vi "Mass_2_2.vi"() -> ()   [LabVIEW 2020]
uses:
  Support/Controls/Cmd_Mouse Popup.ctl
  Support/Controls/Clst_Initialize Input.ctl
  Support/Controls/Clst_Result inspec.ctl
  Support/Controls/Cmd_Var Data IO.ctl
  Variables/Global_Cal Info.vi
  <vilib>/express/express arith-compare/Formula/XNode/ExpressFormulaBlockNode.xnode
panel:
  in  "일괄\n변경":bool=TRUE
  in  "추가문자열":string
  in  "추가단위":string(combo)="mg" caption="단위"
  in  "호칭":string
  out "환산값":string caption="환산값 (g)"
  in  "분동등급":string(combo)
  out "적용?":bool
  in  "다음 버튼":bool
  in  "이전 버튼":bool
  in  "제거":bool
  in  "적용":bool
  in  "추가명목값":string caption="명목값"
  in  "추가":bool
  out "분해능":string caption="저울분해능 (g)"
  out "Data Out":string[][](table)
  out "단위":string
  out "명목질량":string
  in  "기기번호":string
  out "명목값":string
  in  "편심오차":string[][](table) caption="4. 저울 편심오차 시험"
  in  "시험분동밀도":string="8000" caption="분동밀도 (kg/㎤)"
  out "감도분동":string
  out "X=S-T":string[][](table)
  out "공기밀도":string
  out "Header2":string[][](table)
  in  "Measured":string[][](table) caption="3. 저울 지시값"
  out "Weight info":string[][](table) caption="2. 분동식별표기"
  out "Spec":string[][](table)
  in  "시험분동":i32(listbox)=-1
  in  "Spec 변경":bool
  out "제목":string
  out "에러 출력":errorcluster
  out "Condition":string[][](table)
  out "Atm Env":string[][](table) caption="1. 측정환경"
  out "Load?":bool
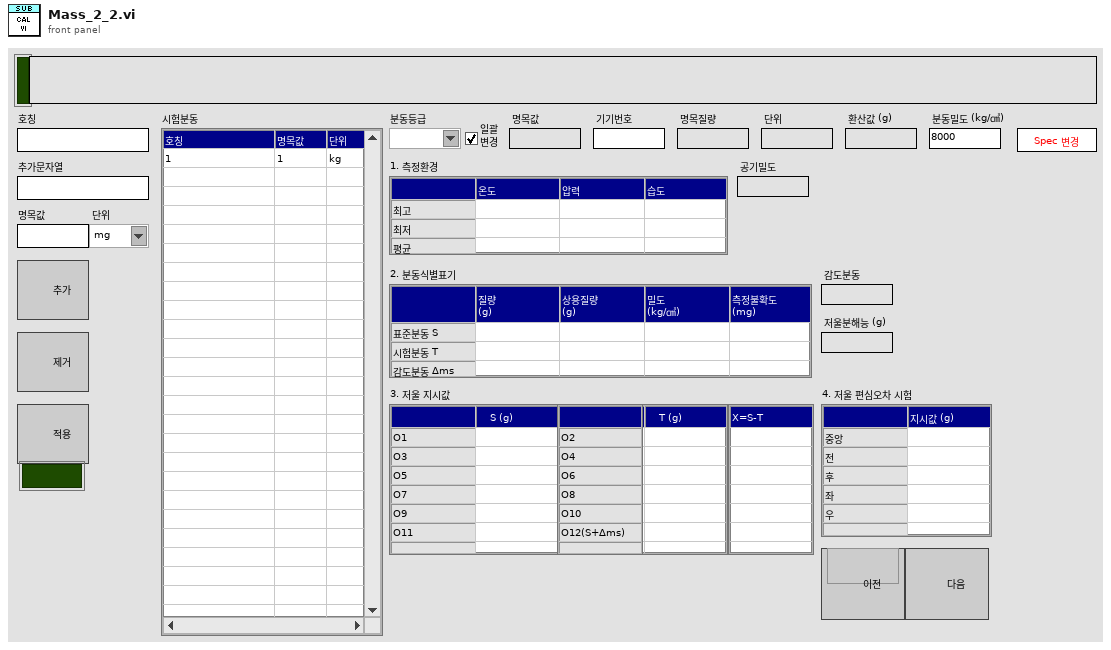
[diagram p1: front panel]
types:
  T1 = typedef "Cmd_Mouse Popup.ctl" = enum16{"활성화", "메뉴선택"}
  T2 = cluster{"Shift":bool, "Ctrl":bool, "Alt":bool, "Cmd":bool, "Opt":bool}
  T3 = typedef "Clst_Initialize Input.ctl" = cluster{"Initialize 1":cluster{"Condition":refnum<vi>[], "Spec":refnum<vi>[], "Measured":refnum<vi>[], "Resolution":refnum<vi>[], "Func_ext":string, "제목":refnum<vi>, "Measured_ADJ":refnum<vi>[]}, "Initialize 2":cluster{"문자열":refnum<vi>[], "콤보박스":refnum<vi>[], "링":refnum<vi>[], "열거형":refnum<vi>[], "테이블":refnum<vi>[], "여러열":refnum<vi>[], "디지털(DBL)":refnum<vi>[], "3D string":refnum<vi>[], "ctrl":refnum<vi>[], "boolean":refnum<vi>[]}}
  T4 = typedef "Cmd_Var Data IO.ctl" = enum16{"Condition", "Condition Default", "Condition_Temp", "Resolution", "Resolution Default", "Resolution Old", "Spec", "Spec Default", "Spec Old", "Spec Temp", "Result", "Result2", "Result3", "Result_Temp", "Result_ADJ", "Result_ADJ2", "STD1", "STD2", "STD3", "STD4", "STD5", "STD Temp", "CMC", "CMC Default"}
  T5 = typedef "Clst_Result inspec.ctl" = cluster{"분해능":string, "문자열 1":string, "문자열 2":string, "숫자형 1":i32, "숫자형 2":i32, "숫자형 3":dbl, "문자배열 1D":string[], "문자배열 2D":string[][], "문자배열 3D":string[][][], "문자배열 4D":string[][][][], "불리언 1D":bool[]}
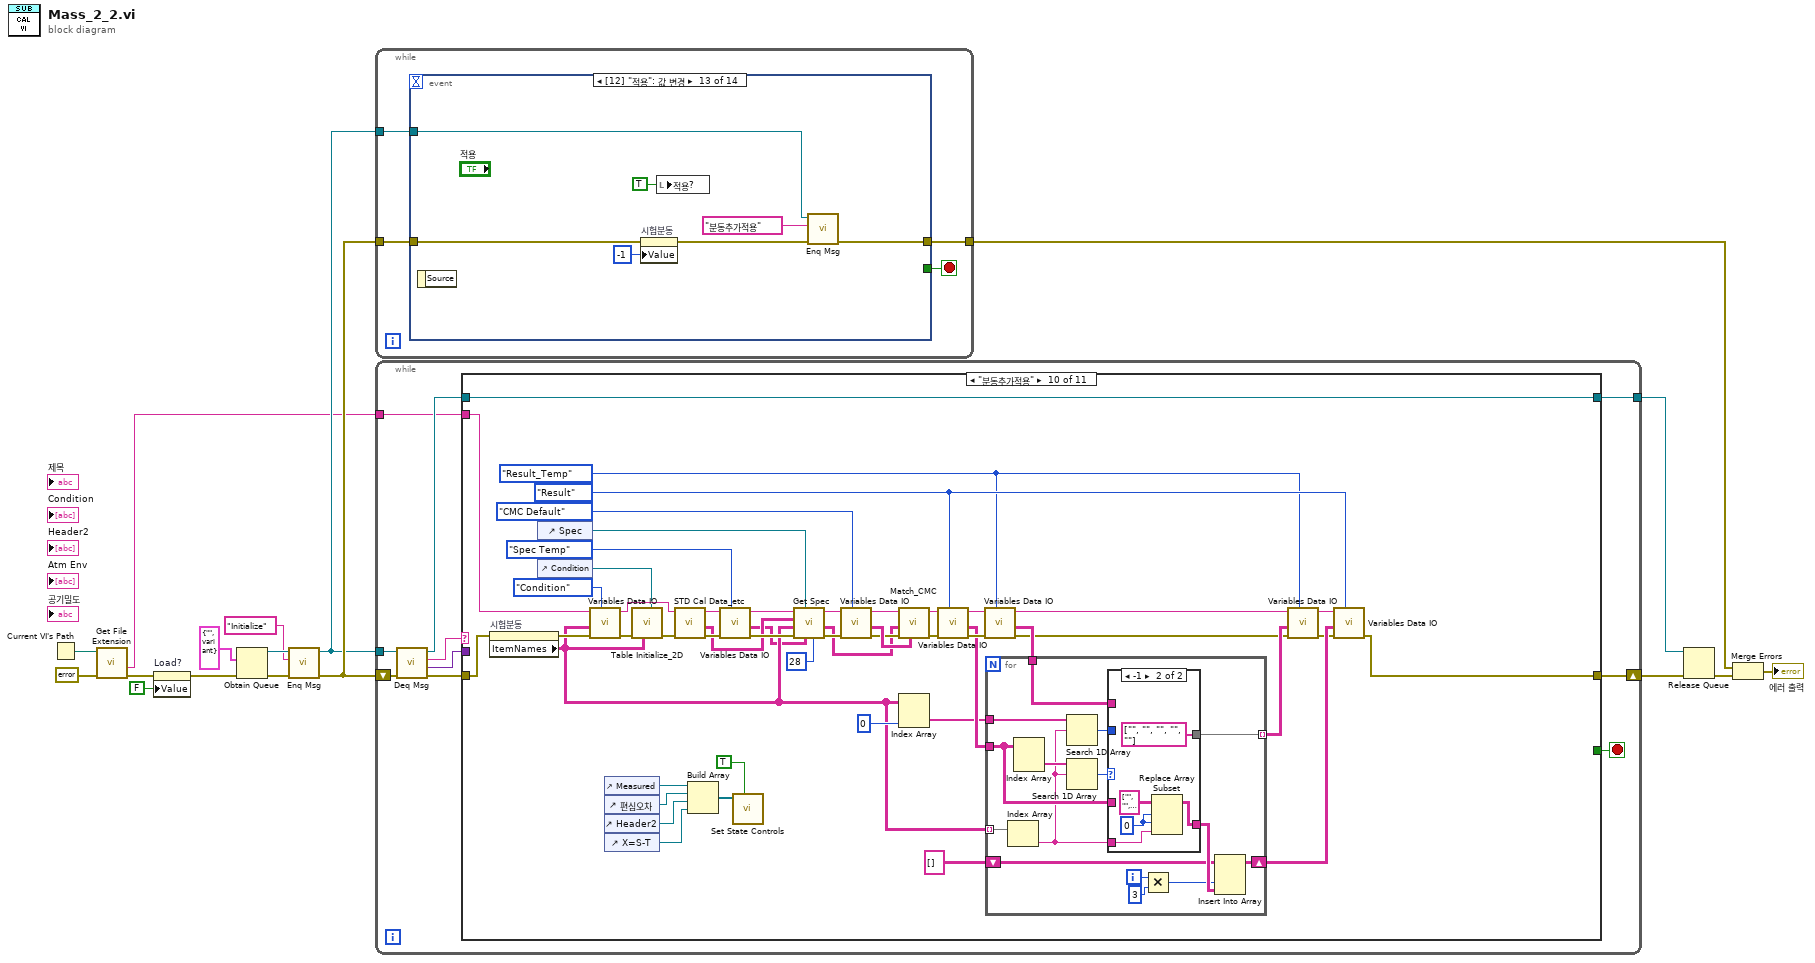
[diagram p0: block diagram]
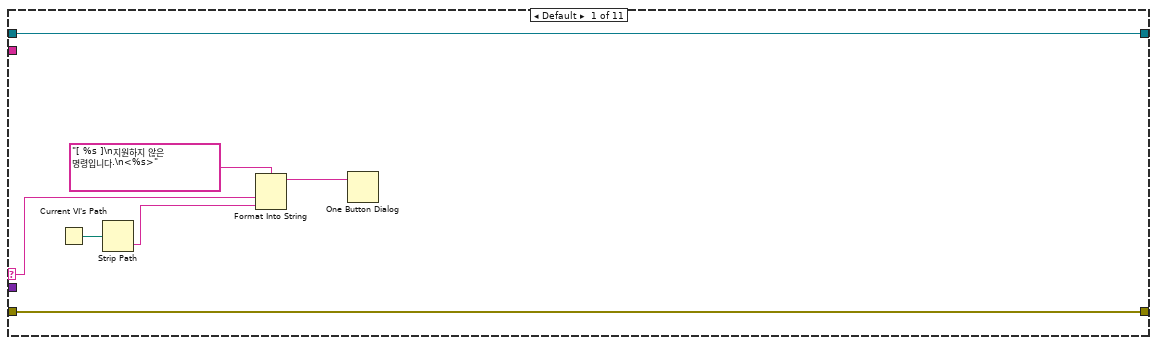
[diagram p2: hidden frame]
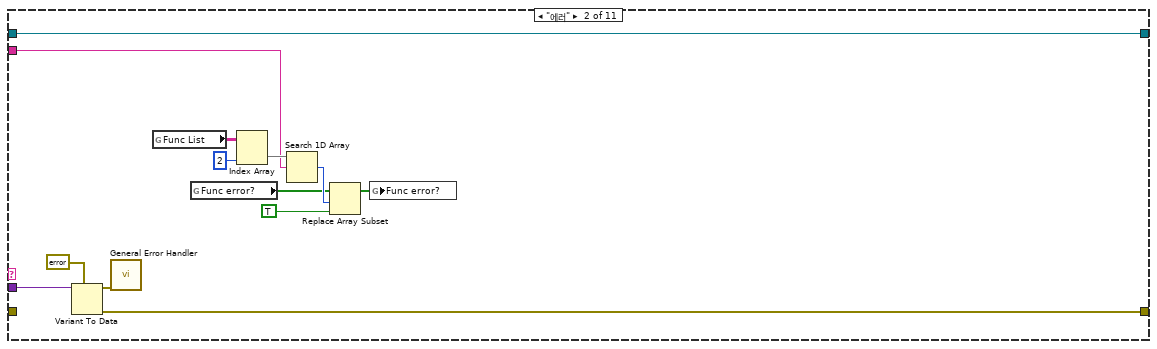
[diagram p3: hidden frame]
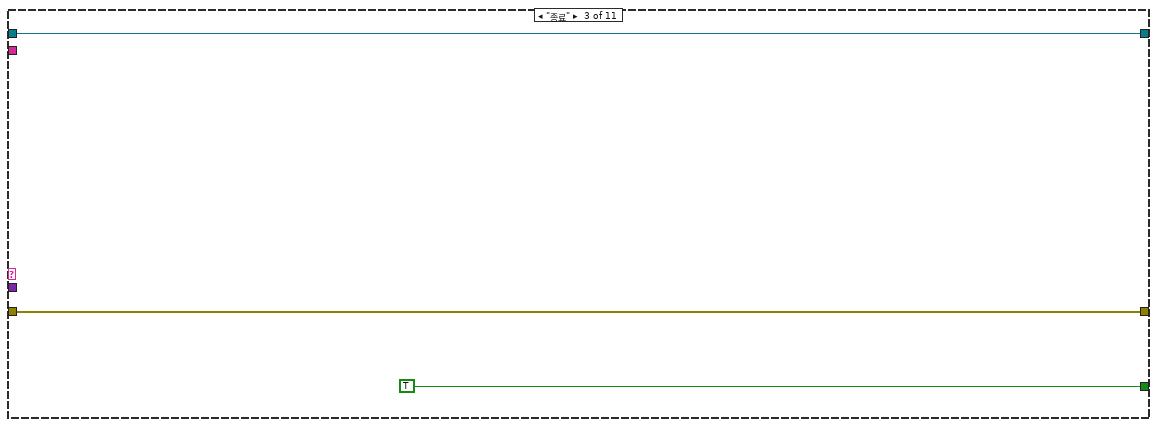
[diagram p4: hidden frame]
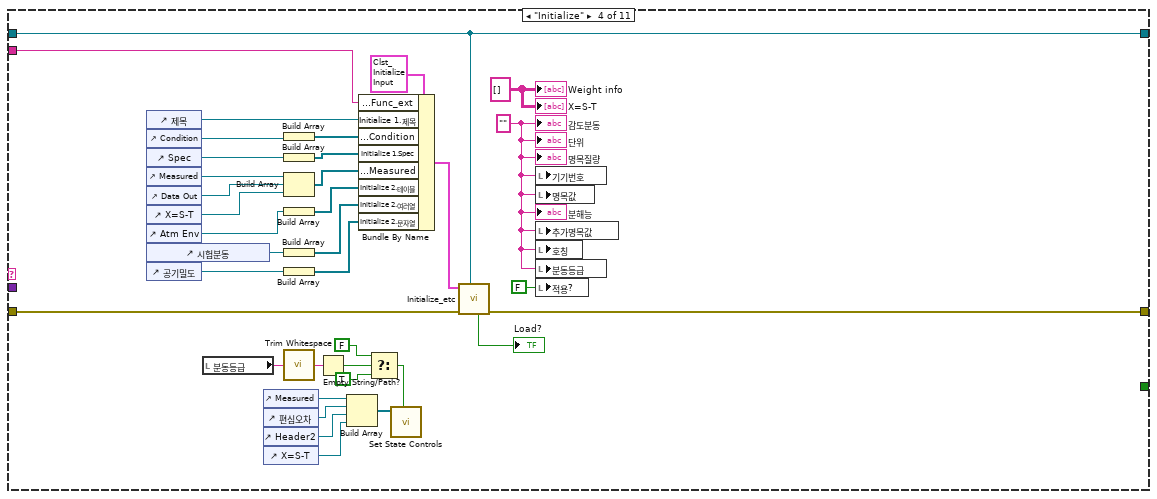
[diagram p5: hidden frame]
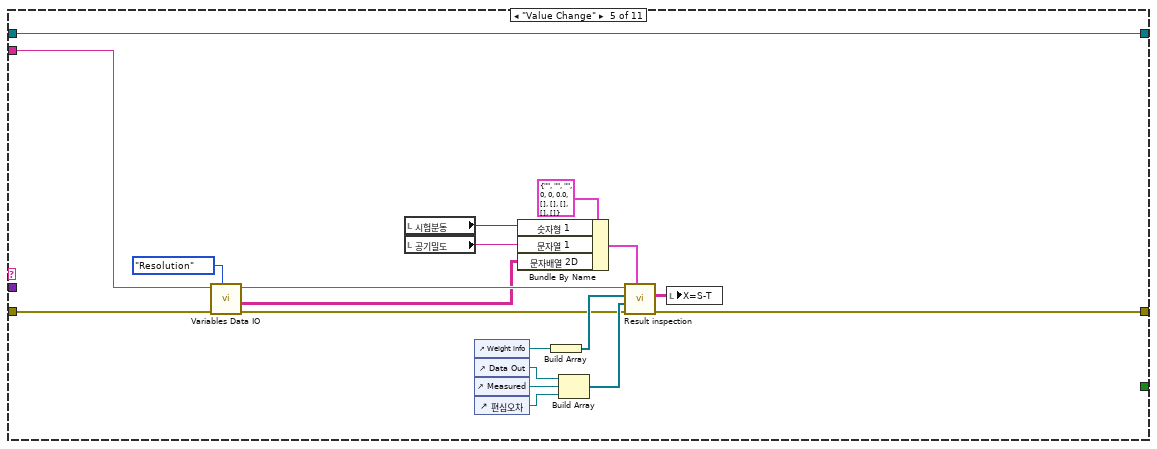
[diagram p6: hidden frame]
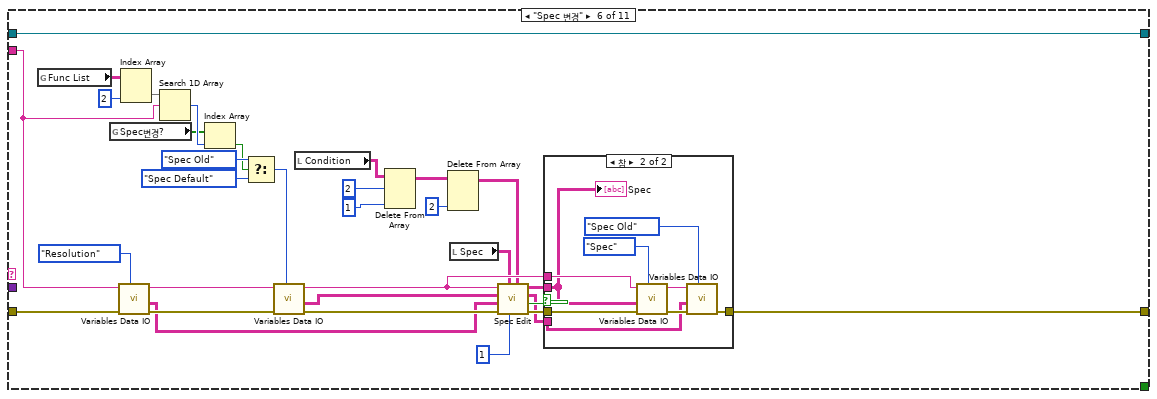
[diagram p7: hidden frame]
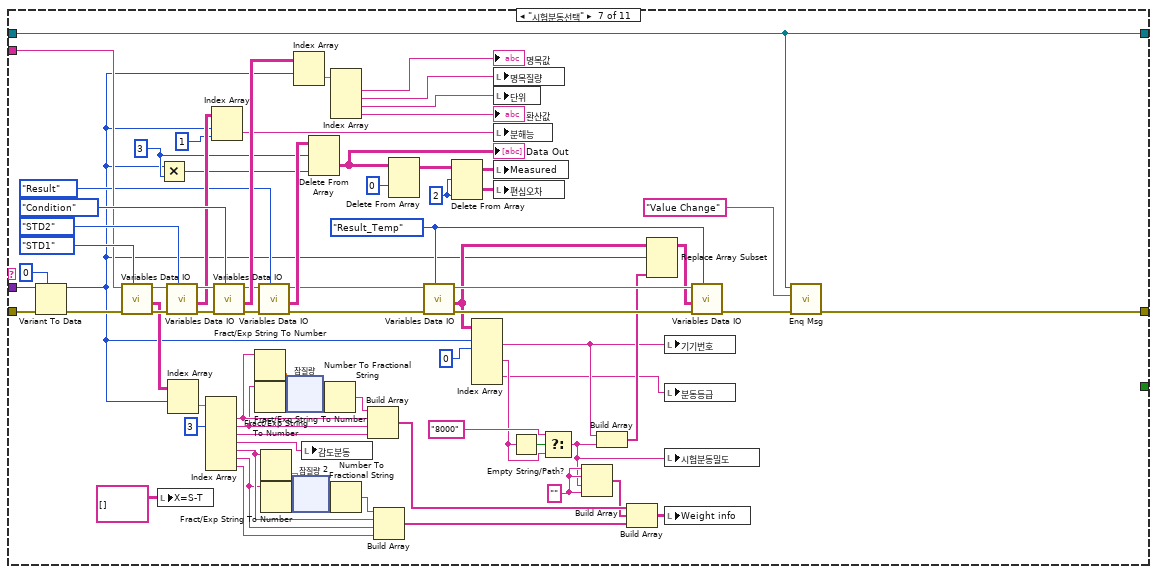
[diagram p9: hidden frame]
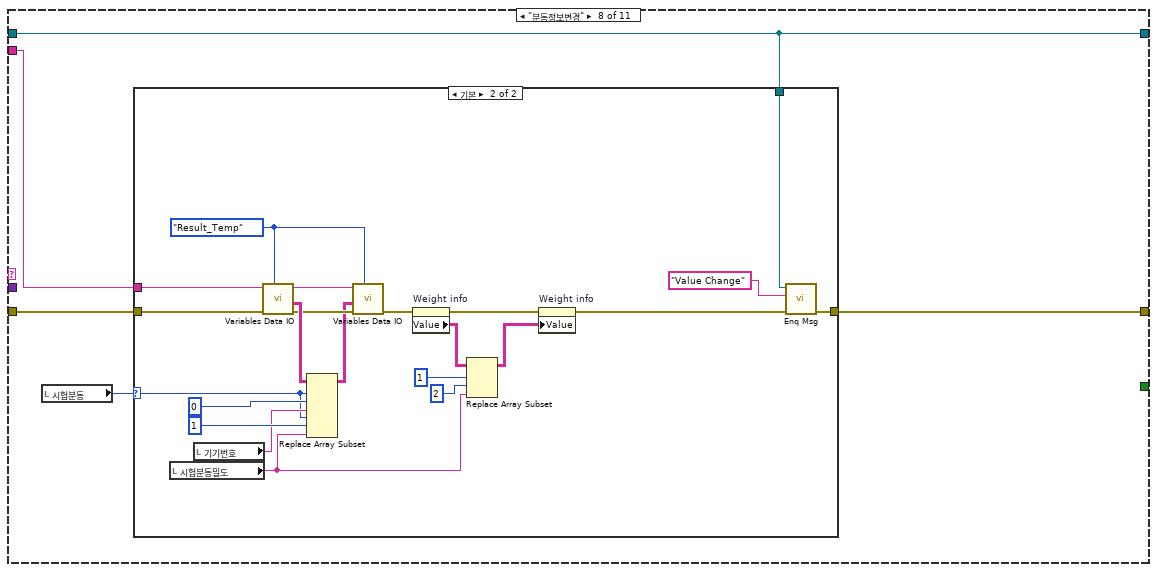
[diagram p10: hidden frame]
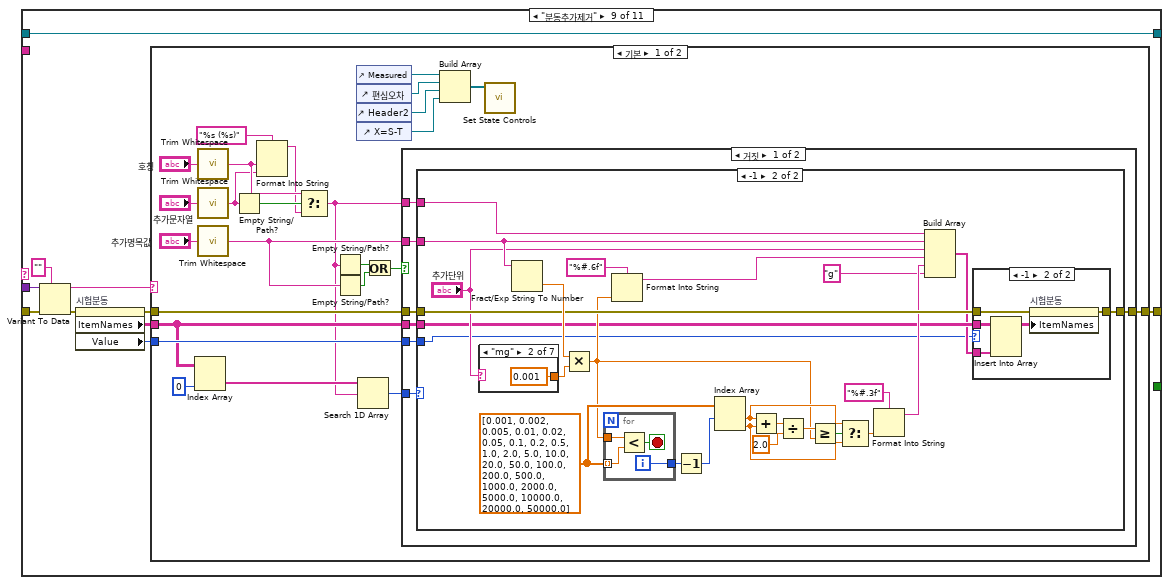
[diagram p12: hidden frame]
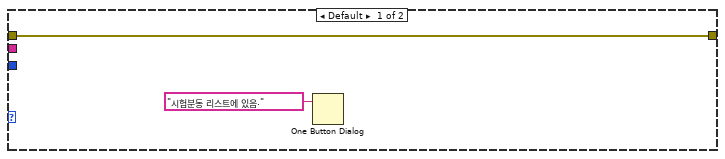
[diagram p13: hidden frame]
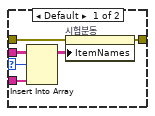
[diagram p14: hidden frame]
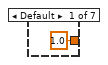
[diagram p15: hidden frame]
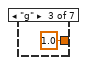
[diagram p16: hidden frame]
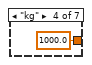
[diagram p17: hidden frame]
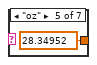
[diagram p18: hidden frame]
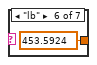
[diagram p19: hidden frame]
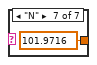
[diagram p20: hidden frame]
diagram:
  n1 = Current VI's Path() -> (path=w5:path)
  n2 = call <vilib>:"Get File Extension.vi"("error in (no error)"=errorcluster {"status"=FALSE, "code"=0, "source"=""} ("에러 상수"), "file"=w5) -> ("error out"=w3:errorcluster, "filename without extension"=w4:string)  [unwired: 5 in, 3 out]
  n3 = property on="Load?" class="Bool (엄격한)"(error in=w3, "Value"=FALSE ("Load?")) -> (error out=w2:errorcluster)  [unwired: 1 in, 1 out]
  n4 = Obtain Queue(element data type=cluster{"메세지":string, "값":variant} {"메세지"="", "값"=variant} ("Message Cluster"), error in (no error)=w2) -> (queue out=w14:refnum<queue>, error out=w16:errorcluster)  [unwired: 3 in, 1 out]
  n5 = call "Enq Msg.vi"("에러 입력(에러 없음)"=w16, "메세지"="Initialize", "큐 입력"=w14) -> ("에러 출력"=w15:errorcluster, "큐 출력"=w12:refnum<queue>)  [unwired: 7 in]
  n6 = while {
    tunnel: w15 -> [w19]
    tunnel: w12 -> [w20]
    tunnel: [w18] -> w9
    stop <- w21 stop-if-true
    n7 = event shown="[12] \"적용\": 값 변경" {
      selector: _ -> [_ _ _ _ _ _ _ _ _ _ _ _ _ _]
      dyn-events: _ -> [_ _ _ _ _ _ _ _ _ _ _ _ _ _]
      timeout: _ -> [_ _ _ _ _ _ _ _ _ _ _ _ _ _]
      tunnel: [w26 _ _ _ _ _ _ _ _ _ _ _ _ _] -> w21
      tunnel: w20 -> [w24 w29 _ w36 _ w49 w58 _ w79 w102 w117 w122 w136 w137]
      tunnel: w19 -> [w25 w30 w33 w41 w48 w51 w60 w72 w81 w96 w119 w129 w134 w139]
      tunnel: [w22 w28 w32 w35 w47 w50 w54 w72 w80 w104 w118 w121 w135 w138] -> w18
      event Panel Close? {
        w26 = TRUE ("버림?")
        n8 = event-data() -> ()  [unwired: 1 in, 1 out]
        n9 = call "Enq Msg.vi"("에러 입력(에러 없음)"=w25, "메세지"="종료", "큐 입력"=w24) -> ("에러 출력"=w22:errorcluster)  [unwired: 7 in, 1 out]
        n10 = event-data("Discard?"=w26) -> ()  [unwired: 1 in, 1 out]
      }
      event "Measured", "편심오차": Value Change {
        n11 = event-data() -> ()  [unwired: 1 in, 3 out]
        n12 = call "Enq Msg.vi"("에러 입력(에러 없음)"=w30, "메세지"="Value Change", "큐 입력"=w29) -> ("에러 출력"=w28:errorcluster)  [unwired: 7 in, 1 out]
      }
      event "Measured", "편심오차": Shortcut Menu Activation? {
        n13 = event-data() -> ("MenuRef"=w31:refnum<k9>)  [unwired: 1 in]
        n14 = call "Mouse PopUp Control.vi"("type"=Cmd_Mouse_Popup."활성화", "error in"=w33, "메뉴 참조"=w31) -> ("error out"=w32:errorcluster)  [unwired: 8 in]
        n15 = event-data() -> ()  [unwired: 2 in, 1 out]
      }
      event "Measured", "편심오차": Shortcut Menu Selection (User) {
        n16 = event-data() -> ("CtlRef"=w39:refnum<vi>, "ItemTag"=w40:string)  [unwired: 1 in]
        n17 = call "Mouse PopUp Control.vi"("type"=Cmd_Mouse_Popup."메뉴선택", "error in"=w41, "아이템 태그"=w40, "Tbl 참조 번호"=w39) -> ("error out"=w37:errorcluster)  [unwired: 7 in]
        n18 = call "Enq Msg.vi"("에러 입력(에러 없음)"=w37, "메세지"="Value Change", "큐 입력"=w36) -> ("에러 출력"=w35:errorcluster)  [unwired: 7 in, 1 out]
      }
      event "Measured", "편심오차", "Condition": Key Down; "Measured", "편심오차", "Condition": Key Repeat {
        n19 = event-data() -> ("PlatMods"=w43:T2, "ScanCode"=w46:i16, "Mods.Num Pad"=w45:bool, "CtlRef"=w44:refnum<vi>)  [unwired: 1 in]
        n20 = call "Cursor Control.vi"("플랫폼 조합키"=w43, "참조"=w44, "Num Pad"=w45, "ScanCode"=w46, "error in"=w48) -> ("error out"=w47:errorcluster)  [unwired: 5 in, 1 out]
      }
      event "Spec 변경": Value Change {
        n21 = event-data() -> ()  [unwired: 1 in, 1 out]
        n22 = call "Enq Msg.vi"("에러 입력(에러 없음)"=w51, "메세지"="Spec 변경", "큐 입력"=w49) -> ("에러 출력"=w50:errorcluster)  [unwired: 7 in, 1 out]
      }
      event "시험분동": Value Change {
        n23 = event-data() -> ()  [unwired: 1 in, 1 out]
        n24 = local read "적용?"() -> (w57:bool)
        n25 = To Variant(anything="시험분동") -> (Variant=w59:variant)
        n26 = Less Than 0?(x="시험분동") -> (x < 0?=w53:bool)
        n27 = case shown="거짓" w57 {
          tunnel: w60 -> [w66 w70]
          tunnel: [w66 w69] -> w55
          tunnel: w59 -> [_ w68]
          tunnel: w58 -> [_ w67]
          frame False {
            n28 = control-ref of="Measured"() -> (w62:refnum<vi>)
            n29 = control-ref of="편심오차"() -> (w61:refnum<vi>)
            n30 = control-ref of="Header2"() -> (w64:refnum<vi>)
            n31 = control-ref of="X=S-T"() -> (w65:refnum<vi>)
            n32 = Build Array(w62, w61, w64, w65) -> (w63:refnum<vi>[])
            n33 = call "Set State Controls.vi"("컨트롤 참조 배열 in"=w63) -> ()  [unwired: 9 in, 2 out]
          }
          frame True {
            n34 = call "Enq Msg.vi"("에러 입력(에러 없음)"=w70, "값"=w68, "메세지"="시험분동선택", "큐 입력"=w67) -> ("에러 출력"=w69:errorcluster)  [unwired: 6 in, 1 out]
          }
        }
        n35 = property on="일괄\n변경" class="Bool (엄격한)"(error in=w55, "Value"=w53) -> (error out=w54:errorcluster)  [unwired: 1 in, 1 out]
      }
      event "시험분동": Drag Ended {
        n36 = event-data() -> ()  [unwired: 1 in, 4 out]
        n37 = control-ref of="Measured"() -> (w74:refnum<vi>)
        n38 = control-ref of="편심오차"() -> (w73:refnum<vi>)
        n39 = control-ref of="Header2"() -> (w76:refnum<vi>)
        n40 = control-ref of="X=S-T"() -> (w77:refnum<vi>)
        n41 = local write "적용?"(FALSE ("적용?")) -> ()
        n42 = Build Array(w74, w73, w76, w77) -> (w75:refnum<vi>[])
        n43 = call "Set State Controls.vi"("컨트롤 참조 배열 in"=w75) -> ()  [unwired: 9 in, 2 out]
      }
      event "시험분동": Double Click {
        n44 = event-data() -> ()  [unwired: 1 in, 1 out]
        n45 = local read "적용?"() -> (w82:bool)
        n46 = case shown="거짓" w82 {
          tunnel: w81 -> [w84 w89]
          tunnel: [w86 w89] -> w80
          tunnel: w79 -> [w85 _]
          frame False {
            n47 = To Variant(anything="제거") -> (Variant=w87:variant)
            n48 = call "Enq Msg.vi"("에러 입력(에러 없음)"=w84, "값"=w87, "메세지"="분동추가제거", "큐 입력"=w85) -> ("에러 출력"=w86:errorcluster)  [unwired: 6 in, 1 out]
          }
          frame True {
          }
        }
      }
      event "이전 버튼", "다음 버튼": Value Change {
        n49 = event-data() -> ()  [unwired: 1 in, 1 out]
        n50 = property on="시험분동" class="MCListbox (엄격한)"(error in=w96) -> (error out=w95:errorcluster, "Value"=w94:i32, "ItemNames"=w93:string[][])  [unwired: 1 in, 1 out]
        n51 = Build Array("이전 버튼", "다음 버튼") -> (w99:bool[])
        n52 = Array Size(array=w93) -> (size(s)=w92:i32[])
        n53 = Boolean Array To Number(Boolean array=w99) -> (number=w98:u32)
        n54 = Index Array(array=w92) -> (element=w91:i32)  [unwired: 1 in]
        n55 = Decrement(x=w91) -> (x-1=w90:i32)
        n56 = case shown="2" w98 {
          tunnel: w94 -> [w106 w110 w116]
          tunnel: [w106 w107 w115] -> w97
          tunnel: w90 -> [_ _ w113]
          frame Default {
          }
          frame 1 {
            n57 = Less Or Equal To 0?(x=w110) -> (x <= 0?=w111:bool)
            n58 = Decrement(x=w110) -> (x-1=w109:i32)
            n59 = Select(t=0, s=w111, f=w109) -> (s? t:f=w107:i32)
          }
          frame 2 {
            n60 = Increment(x=w116) -> (x+1=w114:i32)
            n61 = Less Or Equal?(x=w114, y=w113) -> (x <= y?=w112:bool)
            n62 = Select(t=w114, s=w112, f=w116) -> (s? t:f=w115:i32)
          }
        }
        n63 = local write "시험분동"(w97) -> ()
        n64 = To Variant(anything=w97) -> (Variant=w103:variant)
        n65 = call "Enq Msg.vi"("에러 입력(에러 없음)"=w95, "값"=w103, "메세지"="시험분동선택", "큐 입력"=w102) -> ("에러 출력"=w104:errorcluster)  [unwired: 6 in, 1 out]
      }
      event "기기번호", "시험분동밀도": Value Change {
        n66 = event-data() -> ()  [unwired: 1 in, 3 out]
        n67 = call "Enq Msg.vi"("에러 입력(에러 없음)"=w119, "메세지"="분동정보변경", "큐 입력"=w117) -> ("에러 출력"=w118:errorcluster)  [unwired: 7 in, 1 out]
      }
      event "추가", "제거": Value Change {
        n68 = event-data() -> ("CtlRef"=w128:refnum<vi>)  [unwired: 1 in]
        n69 = property class="Bool"(reference=w128, error in=w129) -> (error out=w124:errorcluster, "Label.Text"=w123:string)  [unwired: 1 out]
        n70 = To Variant(anything=w123) -> (Variant=w125:variant)
        n71 = call "Enq Msg.vi"("에러 입력(에러 없음)"=w124, "값"=w125, "메세지"="분동추가제거", "큐 입력"=w122) -> ("에러 출력"=w121:errorcluster)  [unwired: 6 in, 1 out]
        "적용?" <- FALSE ("적용?")
      }
      event "적용": Value Change {
        n72 = event-data() -> ()  [unwired: 1 in, 1 out]
        n73 = property on="시험분동" class="MCListbox (엄격한)"(error in=w134, "Value"=-1 ("시험분동")) -> (error out=w132:errorcluster)  [unwired: 1 in, 1 out]
        n74 = local write "적용?"(TRUE ("적용?")) -> ()
        n75 = call "Enq Msg.vi"("에러 입력(에러 없음)"=w132, "메세지"="분동추가적용", "큐 입력"=w136) -> ("에러 출력"=w135:errorcluster)  [unwired: 7 in, 1 out]
      }
      event "분동등급": Value Change {
        n76 = event-data() -> ()  [unwired: 1 in, 3 out]
        n77 = call "Enq Msg.vi"("에러 입력(에러 없음)"=w139, "메세지"="분동등급변경", "큐 입력"=w137) -> ("에러 출력"=w138:errorcluster)  [unwired: 7 in, 1 out]
      }
    }
  }
  n78 = while {
    shift-right: [w150] -> w11
    shift-left: w15 -> [w149]
    tunnel: w12 -> [w147]
    tunnel: [w142] -> w10
    tunnel: w4 -> [w141]
    stop <- w143 stop-if-true
    n79 = call "Deq Msg.vi"("에러 입력(에러 없음)"=w149, "큐 입력"=w147) -> ("에러 출력"=w148:errorcluster, "값"=w144:variant, "메세지"=w146:string, "큐 출력"=w145:refnum<queue>)  [unwired: 6 in]
    n80 = case shown="\"분동추가적용\"" w146 {
      selector: w146 -> [w153 _ _ _ _ _ _ _ _ _ _]
      tunnel: w148 -> [w157 _ w173 w178 w214 w254 w347 w372 w403 w525 w582]
      tunnel: [w157 w167 w173 w196 w224 w258 w274 w371 w397 w514 w577] -> w150
      tunnel: w145 -> [w156 w166 w171 w195 w228 w260 w273 w368 w405 w544 w593]
      tunnel: w144 -> [_ w168 _ _ _ _ w346 _ w402 _ _]
      tunnel: [_ _ TRUE ("버림?") _ _ _ _ _ _ _ _] -> w143
      tunnel: [w156 w166 w171 w195 w228 w260 w273 w368 w405 w544 w593] -> w142
      tunnel: w141 -> [_ w158 _ w199 w212 w236 w324 w370 _ w524 w581]
      frame Default {
        n81 = Current VI's Path() -> (path=w152:path)
        n82 = Strip Path(path=w152) -> (name=w151:string)  [unwired: 1 out]
        n83 = Format Into String(format string="[ %s ]\n지원하지 않은 명령입니다.\n<%s>" ("메시지"), w153, w151) -> (resulting string=w154:string)  [unwired: 2 in, 1 out]
        n84 = One Button Dialog(message=w154) -> ()  [unwired: 1 in, 1 out]
      }
      frame "에러" {
        n85 = Variant To Data(type=errorcluster {"status"=FALSE, "code"=0, "source"=""} ("에러 출력"), Variant=w168) -> (data=w170:errorcluster, error out=w167:errorcluster)  [unwired: 1 in]
        n86 = call <vilib>:"General Error Handler.vi"("error in (no error)"=w170) -> ()  [unwired: 10 in, 5 out]
        n87 = global read "Global_Cal Info.vi" "Func List"() -> (w160:string[][])
        n88 = global read "Global_Cal Info.vi" "Func error?"() -> (w163:bool[])
        n89 = Index Array(array=w160, index (col)=2 ("비활성화된 인덱스 (열)")) -> (element=w161:string[])  [unwired: 1 in]
        n90 = Search 1D Array(1D array=w161, element=w158) -> (index of element=w164:i32)  [unwired: 1 in]
        n91 = Replace Array Subset(array=w163, new element=TRUE ("새 원소/부분배열"), index=w164) -> (w165:bool[])
        n92 = global write "Global_Cal Info.vi" "Func error?"(w165) -> ()
      }
      frame "종료" {
      }
      frame "Initialize" {
        w194 = string[][] [] ("Weight info")
        w175 = "" ("감도 분동")
        n93 = control-ref of="제목"() -> (w202:refnum<vi>)
        n94 = control-ref of="Condition"() -> (w207:refnum<vi>)
        n95 = control-ref of="Spec"() -> (w201:refnum<vi>)
        n96 = control-ref of="Measured"() -> (w204:refnum<vi>)
        n97 = control-ref of="Data Out"() -> (w177:refnum<vi>)
        n98 = control-ref of="X=S-T"() -> (w176:refnum<vi>)
        n99 = control-ref of="Atm Env"() -> (w190:refnum<vi>)
        n100 = control-ref of="시험분동"() -> (w198:refnum<vi>)
        n101 = control-ref of="공기밀도"() -> (w192:refnum<vi>)
        n102 = local read "분동등급"() -> (w184:string)
        n103 = control-ref of="Measured"() -> (w186:refnum<vi>)
        n104 = control-ref of="편심오차"() -> (w187:refnum<vi>)
        n105 = control-ref of="Header2"() -> (w188:refnum<vi>)
        n106 = control-ref of="X=S-T"() -> (w189:refnum<vi>)
        n107 = Build Array(w207) -> (w206:refnum<vi>[])
        n108 = Build Array(w201) -> (w200:refnum<vi>[])
        n109 = Build Array(w204, w177, w176) -> (w205:refnum<vi>[])
        n110 = Build Array(w190) -> (w203:refnum<vi>[])
        n111 = Build Array(w198) -> (w197:refnum<vi>[])
        n112 = Build Array(w192) -> (w191:refnum<vi>[])
        n113 = call <vilib>:"Trim Whitespace.vi"("string"=w184) -> ("trimmed string"=w183:string)  [unwired: 1 in]
        n114 = Empty String/Path?(string/path=w183) -> (empty?=w182:bool)
        n115 = Build Array(w186, w187, w188, w189) -> (w185:refnum<vi>[])
        n116 = Bundle By Name(cluster=T3 {"Initialize 1"={"Condition"=[], "Spec"=[], "Measured"=[], "Resolution"=[], "Func_ext"="", "제목"=refnum, "Measured_ADJ"=[]}, "Initialize 2"={"문자열"=[], "콤보박스"=[], "링"=[], "열거형"=[], "테이블"=[], "여러열"=[], "디지털(DBL)"=[], "3D string"=[], "ctrl"=[], "boolean"=[]}} ("입력 클러스터"), "Initialize 1.Func_ext"=w199, "Initialize 1.제목"=w202, "Initialize 1.Condition"=w206, "Initialize 1.Spec"=w200, "Initialize 1.Measured"=w205, "Initialize 2.테이블"=w203, "Initialize 2.여러열"=w197, "Initialize 2.문자열"=w191) -> (w208:T3)
        n117 = Select(t=FALSE, s=w182, f=TRUE) -> (s? t:f=w179:bool)
        n118 = call "Set State Controls.vi"("활성화 (F)"=w179, "컨트롤 참조 배열 in"=w185) -> ()  [unwired: 8 in, 2 out]
        n119 = call "Initialize_etc.vi"("큐 입력"=w195, "error in"=w178, "입력 클러스터"=w208) -> ("error out"=w196:errorcluster, "Load?"=→"Load?":bool)  [unwired: 6 in, 1 out]
        n120 = local write "기기번호"(w175) -> ()
        n121 = local write "명목값"(w175) -> ()
        n122 = local write "추가명목값"(w175) -> ()
        n123 = local write "호칭"(w175) -> ()
        n124 = local write "분동등급"(w175) -> ()
        n125 = local write "적용?"(FALSE ("적용?")) -> ()
        "감도분동" <- w175
        "Weight info" <- w194
        "단위" <- w175
        "명목질량" <- w175
        "X=S-T" <- w194
        "분해능" <- w175
      }
      frame "Value Change" {
        n126 = call "Variables Data IO.vi"("Select"=Cmd_Var_Data_IO."Resolution", "error in"=w214, "Func_ext"=w212) -> ("error out"=w213:errorcluster, "Data Out"=w210:string[][], "Func_ext Out"=w211:string)  [unwired: 6 in]
        n127 = local read "시험분동"() -> (w221:i32)
        n128 = local read "공기밀도"() -> (w220:string)
        n129 = control-ref of="Weight info"() -> (w223:refnum<vi>)
        n130 = control-ref of="Data Out"() -> (w217:refnum<vi>)
        n131 = control-ref of="Measured"() -> (w216:refnum<vi>)
        n132 = control-ref of="편심오차"() -> (w218:refnum<vi>)
        n133 = Bundle By Name(cluster=T5 {"분해능"="", "문자열 1"="", "문자열 2"="", "숫자형 1"=0, "숫자형 2"=0, "숫자형 3"=0.0, "문자배열 1D"=[], "문자배열 2D"=[], "문자배열 3D"=[], "문자배열 4D"=[], "불리언 1D"=[]} ("입력 클러스터"), "숫자형 1"=w221, "문자열 1"=w220, "문자배열 2D"=w210) -> (w225:T5)
        n134 = Build Array(w223) -> (w227:refnum<vi>[])
        n135 = Build Array(w217, w216, w218) -> (w222:refnum<vi>[])
        n136 = call "Result inspection.vi"("입력 클러스터"=w225, "error in"=w213, "Ref. Data (excluded)"=w222, "Ref. Data (Inspection)"=w227, "Func ext"=w211) -> ("error out"=w224:errorcluster, "Data (spec 미적용)"=w219:string[][])  [unwired: 3 in, 2 out]
        n137 = local write "X=S-T"(w219) -> ()
      }
      frame "Spec 변경" {
        n138 = global read "Global_Cal Info.vi" "Func List"() -> (w241:string[][])
        n139 = global read "Global_Cal Info.vi" "Spec변경?"() -> (w237:bool[])
        n140 = call "Variables Data IO.vi"("Select"=Cmd_Var_Data_IO."Resolution", "error in"=w254, "Func_ext"=w236) -> ("error out"=w253:errorcluster, "Data Out"=w247:string[][], "Func_ext Out"=w252:string)  [unwired: 6 in]
        n141 = Index Array(array=w241, index (col)=2 ("비활성화된 인덱스 (열)")) -> (element=w239:string[])  [unwired: 1 in]
        n142 = Search 1D Array(1D array=w239, element=w236) -> (index of element=w238:i32)  [unwired: 1 in]
        n143 = Index Array(array=w237, index=w238) -> (element=w242:bool)
        n144 = Select(t=Cmd_Var_Data_IO."Spec Old" ("Select"), s=w242, f=Cmd_Var_Data_IO."Spec Default" ("Select")) -> (s? t:f=w235:T4)
        n145 = call "Variables Data IO.vi"("Select"=w235, "error in"=w253, "Func_ext"=w252) -> ("error out"=w255:errorcluster, "Data Out"=w246:string[][], "Func_ext Out"=w248:string)  [unwired: 6 in]
        n146 = local read "Condition"() -> (w234:string[][])
        n147 = Delete From Array(array=w234, length=2 ("길이"), index (col)=1 ("비활성화된 인덱스 (열)")) -> (array with subset deleted=w231:string[][])  [unwired: 1 in, 1 out]
        n148 = Delete From Array(array=w231, index (col)=2 ("비활성화된 인덱스 (열)")) -> (array with subset deleted=w230:string[][])  [unwired: 2 in, 1 out]
        n149 = local read "Spec"() -> (w245:string[][])
        n150 = call "Spec Edit.vi"("Condition"=w230, "열번호(기준값)"=1 ("기준열(0)"), "Spec Value"=w245, "에러 입력(에러 없음)"=w255, "Resolution"=w247, "Spec Default"=w246, "Func_ext"=w248) -> ("에러 출력"=w259:errorcluster, "변경?"=w256:bool, "Spec Default out"=w250:string[][], "Spec 출력"=w257:string[][])  [unwired: 1 in]
        n151 = case shown="참" w256 {
          tunnel: w259 -> [w261 w269]
          tunnel: [w261 w265] -> w258
          tunnel: w257 -> [_ w267]
          tunnel: w248 -> [_ w268]
          tunnel: w250 -> [_ w263]
          frame False {
          }
          frame True {
            n152 = call "Variables Data IO.vi"("Select"=Cmd_Var_Data_IO."Spec", "error in"=w269, "Data In"=w267, "Func_ext"=w268) -> ("error out"=w266:errorcluster, "Func_ext Out"=w264:string)  [unwired: 5 in, 1 out]
            n153 = call "Variables Data IO.vi"("Select"=Cmd_Var_Data_IO."Spec Old", "error in"=w266, "Data In"=w263, "Func_ext"=w264) -> ("error out"=w265:errorcluster)  [unwired: 5 in, 2 out]
            "Spec" <- w267
          }
        }
      }
      frame "시험분동선택" {
        w285 = 2 ("비활성화된 인덱스 (열)")
        w294 = Cmd_Var_Data_IO."Result_Temp" ("Select")
        w301 = "" ("원소")
        w303 = 3 ("길이")
        n154 = Variant To Data(error in=w347, type=0, Variant=w346) -> (data=w283:i32, error out=w323:errorcluster)
        n155 = call "Variables Data IO.vi"("Select"=Cmd_Var_Data_IO."STD1", "error in"=w323, "Func_ext"=w324) -> ("error out"=w331:errorcluster, "Data Out"=w321:string[][], "Func_ext Out"=w330:string)  [unwired: 6 in]
        n156 = local write "X=S-T"(string[][] [] ("X=S-T")) -> ()
        n157 = Multiply(x=w283, y=w303) -> (x*y=w302:i32)
        n158 = call "Variables Data IO.vi"("Select"=Cmd_Var_Data_IO."STD2", "error in"=w331, "Func_ext"=w330) -> ("error out"=w322:errorcluster, "Data Out"=w310:string[][], "Func_ext Out"=w311:string)  [unwired: 6 in]
        n159 = Index Array(array=w321, index (row)=w283) -> (element=w320:string[])  [unwired: 1 in]
        n160 = Index Array(array=w320, index #1=3 ("인덱스")) -> (element #1=w318:string, element #2=w317:string, element #3=w316:string, element #4=w315:string, element #5=w314:string, element #6=w313:string, element #7=w312:string)  [unwired: 6 in]
        n161 = Index Array(array=w310, index (row)=w283, index (col)=1 ("비활성화된 인덱스 (열)")) -> (element=w308:string)
        n162 = call "Variables Data IO.vi"("Select"=Cmd_Var_Data_IO."Condition", "error in"=w322, "Func_ext"=w311) -> ("error out"=w307:errorcluster, "Data Out"=w328:string[][], "Func_ext Out"=w306:string)  [unwired: 6 in]
        n163 = Fract/Exp String To Number(string=w318) -> (number=w342:dbl)  [unwired: 3 in, 1 out]
        n164 = Fract/Exp String To Number(string=w317) -> (number=w341:dbl)  [unwired: 3 in, 1 out]
        n165 = call "Variables Data IO.vi"("Select"=Cmd_Var_Data_IO."Result", "error in"=w307, "Func_ext"=w306) -> ("error out"=w298:errorcluster, "Data Out"=w304:string[][], "Func_ext Out"=w296:string)  [unwired: 6 in]
        n166 = Fract/Exp String To Number(string=w314) -> (number=w337:dbl)  [unwired: 3 in, 1 out]
        n167 = Fract/Exp String To Number(string=w313) -> (number=w336:dbl)  [unwired: 3 in, 1 out]
        n168 = xnode "참질량"("mc"=w342, "d"=w341) -> ("결과"=w340:dbl)  [unwired: 1 in, 1 out]
        n169 = xnode "참질량 2"("mc"=w337, "d"=w336) -> ("결과"=w335:dbl)  [unwired: 1 in, 1 out]
        n170 = Index Array(array=w328, index (row)=w283) -> (element=w327:string[])  [unwired: 1 in]
        n171 = local write "감도분동"(w315) -> ()
        n172 = Delete From Array(array=w304, length=w303, index (col)=w302) -> (deleted portion=w290:string[][])  [unwired: 1 in, 1 out]
        "Data Out" <- w290
        n173 = Number To Fractional String(number=w340) -> (F-format string=w339:string)  [unwired: 3 in]
        n174 = Index Array(array=w327) -> (element #1=→"명목값":string, element #2=w326:string, element #3=w325:string, element #4=→"환산값":string)  [unwired: 4 in]
        n175 = Number To Fractional String(number=w335) -> (F-format string=w334:string)  [unwired: 3 in]
        n176 = Build Array(w339, w318, w317, w316) -> (w338:string[])
        n177 = Build Array(w334, w314, w313, w312) -> (w333:string[])
        n178 = Delete From Array(array=w290, index (row)=0 ("인덱스 (행)")) -> (array with subset deleted=w288:string[][])  [unwired: 2 in, 1 out]
        n179 = call "Variables Data IO.vi"("Select"=w294, "error in"=w298, "Func_ext"=w296) -> ("error out"=w297:errorcluster, "Data Out"=w284:string[][], "Func_ext Out"=w295:string)  [unwired: 6 in]
        n180 = Delete From Array(array=w288, length=w285, index (col)=w285) -> (deleted portion=w286:string[][], array with subset deleted=w287:string[][])  [unwired: 1 in]
        n181 = Index Array(array=w284, index (row) #1=w283, index (col) #1=0 ("비활성화된 인덱스 (열)")) -> (element #1=w277:string, element #2=w278:string, element #3=w271:string)  [unwired: 4 in]
        n182 = local write "명목질량"(w326) -> ()
        n183 = local write "단위"(w325) -> ()
        n184 = local write "분해능"(w308) -> ()
        n185 = local write "Measured"(w287) -> ()
        n186 = local write "편심오차"(w286) -> ()
        n187 = Empty String/Path?(string/path=w278) -> (empty?=w281:bool)
        n188 = Select(t="8000" ("원소"), s=w281, f=w278) -> (s? t:f=w279:string)
        n189 = Build Array(w301, w301, w279, w301) -> (w300:string[])
        n190 = Build Array(w277, w279) -> (w293:string[])
        n191 = Build Array(w338, w300, w333) -> (w332:string[][])
        n192 = Replace Array Subset(array=w284, new element=w293, index (row)=w283) -> (w292:string[][])  [unwired: 1 in]
        n193 = local write "기기번호"(w277) -> ()
        n194 = local write "분동등급"(w271) -> ()
        n195 = local write "시험분동밀도"(w279) -> ()
        n196 = local write "Weight info"(w332) -> ()
        n197 = call "Variables Data IO.vi"("Select"=w294, "error in"=w297, "Data In"=w292, "Func_ext"=w295) -> ("error out"=w275:errorcluster)  [unwired: 5 in, 2 out]
        n198 = call "Enq Msg.vi"("에러 입력(에러 없음)"=w275, "메세지"="Value Change", "큐 입력"=w273) -> ("에러 출력"=w274:errorcluster)  [unwired: 7 in, 1 out]
      }
      frame "분동정보변경" {
        n199 = local read "시험분동"() -> (w369:i32)
        n200 = case shown="기본" w369 {
          selector: w369 -> [_ w374]
          tunnel: w372 -> [w373 w394]
          tunnel: [w373 w386] -> w371
          tunnel: w370 -> [_ w395]
          tunnel: w368 -> [_ w385]
          frame -1 {
          }
          frame Default {
            w388 = Cmd_Var_Data_IO."Result_Temp" ("Select")
            n201 = local read "시험분동밀도"() -> (w379:string)
            n202 = local read "기기번호"() -> (w375:string)
            n203 = call "Variables Data IO.vi"("Select"=w388, "error in"=w394, "Func_ext"=w395) -> ("error out"=w390:errorcluster, "Data Out"=w393:string[][], "Func_ext Out"=w389:string)  [unwired: 6 in]
            n204 = Replace Array Subset(array=w393, new element #1=w375, index (row) #1=w374, index (col) #1=0 ("비활성화된 인덱스 (열)"), new element #2=w379, index (row) #2=w374, index (col) #2=1 ("비활성화된 인덱스 (열)")) -> (w387:string[][])
            n205 = call "Variables Data IO.vi"("Select"=w388, "error in"=w390, "Data In"=w387, "Func_ext"=w389) -> ("error out"=w383:errorcluster)  [unwired: 5 in, 2 out]
            n206 = property on="Weight info" class="Tbl (엄격한)"(error in=w383) -> (error out=w378:errorcluster, "Value"=w382:string[][])  [unwired: 1 in, 1 out]
            n207 = Replace Array Subset(array=w382, new element=w379, index (row)=1 ("인덱스 (행)"), index (col)=2 ("비활성화된 인덱스 (열)")) -> (w377:string[][])
            n208 = property on="Weight info" class="Tbl (엄격한)"(error in=w378, "Value"=w377) -> (error out=w376:errorcluster)  [unwired: 1 in, 1 out]
            n209 = call "Enq Msg.vi"("에러 입력(에러 없음)"=w376, "메세지"="Value Change", "큐 입력"=w385) -> ("에러 출력"=w386:errorcluster)  [unwired: 7 in, 1 out]
          }
        }
      }
      frame "분동추가제거" {
        n210 = Variant To Data(error in=w403, type="", Variant=w402) -> (data=w401:string, error out=w400:errorcluster)
        n211 = property on="시험분동" class="MCListbox (엄격한)"(error in=w400) -> (error out=w399:errorcluster, "ItemNames"=w398:string[][], "Value"=w396:i32)  [unwired: 1 in, 1 out]
        n212 = case shown="기본" w401 {
          tunnel: w399 -> [w430 w494]
          tunnel: w398 -> [w422 w492]
          tunnel: [w429 w493] -> w397
          tunnel: w396 -> [w428 w491]
          frame Default {
            n213 = Index Array(array=w422, index (col)=0 ("비활성화된 인덱스 (열)")) -> (element=w420:string[])  [unwired: 1 in]
            n214 = call <vilib>:"Trim Whitespace.vi"("string"="호칭") -> ("trimmed string"=w415:string)  [unwired: 1 in]
            n215 = call <vilib>:"Trim Whitespace.vi"("string"="추가문자열") -> ("trimmed string"=w414:string)  [unwired: 1 in]
            n216 = call <vilib>:"Trim Whitespace.vi"("string"="추가명목값") -> ("trimmed string"=w423:string)  [unwired: 1 in]
            n217 = Empty String/Path?(string/path=w414) -> (empty?=w416:bool)
            n218 = Format Into String(format string="%s (%s)" ("포맷 문자열"), w415, w414) -> (resulting string=w412:string)  [unwired: 2 in, 1 out]
            n219 = Select(t=w415, s=w416, f=w412) -> (s? t:f=w411:string)
            n220 = Empty String/Path?(string/path=w411) -> (empty?=w426:bool)
            n221 = Empty String/Path?(string/path=w423) -> (empty?=w425:bool)
            n222 = control-ref of="Measured"() -> (w409:refnum<vi>)
            n223 = control-ref of="편심오차"() -> (w410:refnum<vi>)
            n224 = control-ref of="Header2"() -> (w407:refnum<vi>)
            n225 = control-ref of="X=S-T"() -> (w406:refnum<vi>)
            n226 = Search 1D Array(1D array=w420, element=w411) -> (index of element=w419:i32)  [unwired: 1 in]
            n227 = Or(x=w426, y=w425) -> (x .or. y?=w424:bool)
            n228 = case shown="거짓" w424 {
              tunnel: w430 -> [w437 w489]
              tunnel: [w436 w489] -> w429
              tunnel: w411 -> [w435 _]
              tunnel: w423 -> [w434 _]
              tunnel: w422 -> [w433 _]
              tunnel: w428 -> [w432 _]
              tunnel: w419 -> [w431 _]
              frame False {
                n229 = case shown="-1" w431 {
                  tunnel: w437 -> [w439 w452]
                  tunnel: [w439 w451] -> w436
                  tunnel: w435 -> [_ w450]
                  tunnel: w434 -> [_ w449]
                  tunnel: w433 -> [_ w442]
                  tunnel: w432 -> [_ w440]
                  frame Default {
                    n230 = One Button Dialog(message="시험분동 리스트에 있음." ("메시지")) -> ()  [unwired: 1 in, 1 out]
                  }
                  frame -1 {
                    w463 = dbl[] [0.001, 0.002, 0.005, 0.01, 0.02, 0.05, 0.1, 0.2, 0.5, 1.0, 2.0, 5.0, 10.0, 20.0, 50.0, 100.0, 200.0, 500.0, 1000.0, 2000.0, 5000.0, 10000.0, 20000.0, 50000.0]
                    n231 = case shown="\"mg\"" "추가단위" {
                      tunnel: [1.0 0.001 1.0 1000.0 28.34952 453.5924 101.9716] -> w464
                      frame Default {
                      }
                      frame "mg" {
                      }
                      frame "g" {
                      }
                      frame "kg" {
                      }
                      frame "oz" {
                      }
                      frame "lb" {
                      }
                      frame "N" {
                      }
                    }
                    n232 = Fract/Exp String To Number(string=w449) -> (number=w465:dbl)  [unwired: 3 in, 1 out]
                    n233 = Multiply(x=w465, y=w464) -> (x*y=w445:dbl)
                    n234 = for {
                      tunnel: w445 -> [w480]
                      tunnel: w463 -> [w479] mode=indexing
                      tunnel: [w477] -> w462
                      i -> [w477]
                      stop <- w478 stop-if-true
                      n235 = Less?(x=w480, y=w479) -> (x < y?=w478:bool)
                    }
                    n236 = Format Into String(format string="%#.6f" ("포맷 문자열"), w445) -> (resulting string=w446:string)  [unwired: 2 in, 1 out]
                    n237 = Decrement(x=w462) -> (x-1=w461:i32)
                    n238 = Index Array(array=w463, index #1=w461) -> (element #1=w456:dbl, element #2=w455:dbl)  [unwired: 1 in]
                    n239 = Add(x=w456, y=w455) -> (x+y=w460:dbl)
                    n240 = Divide(x=w460, y=2.0) -> (x/y=w458:dbl)
                    n241 = Greater Or Equal?(x=w458, y=w445) -> (x >= y?=w457:bool)
                    n242 = Select(t=w456, s=w457, f=w455) -> (s? t:f=w453:dbl)
                    n243 = Format Into String(format string="%#.3f" ("포맷 문자열"), w453) -> (resulting string=w444:string)  [unwired: 2 in, 1 out]
                    n244 = Build Array(w450, w449, "추가단위", w446, w444, "g" ("원소")) -> (w441:string[])
                    n245 = case shown="-1" w440 {
                      selector: w440 -> [w466 _]
                      tunnel: w452 -> [w471 w476]
                      tunnel: [w470 w475] -> w451
                      tunnel: w442 -> [w469 w474]
                      tunnel: w441 -> [w468 w473]
                      frame Default {
                        n246 = Insert Into Array(array=w469, index (row)=w466, new element=w468) -> (w467:string[][])  [unwired: 1 in]
                        n247 = property on="시험분동" class="MCListbox (엄격한)"(error in=w471, "ItemNames"=w467) -> (error out=w470:errorcluster)  [unwired: 1 in, 1 out]
                      }
                      frame -1 {
                        n248 = Insert Into Array(array=w474, new element=w473) -> (w472:string[][])  [unwired: 2 in]
                        n249 = property on="시험분동" class="MCListbox (엄격한)"(error in=w476, "ItemNames"=w472) -> (error out=w475:errorcluster)  [unwired: 1 in, 1 out]
                      }
                    }
                  }
                }
              }
              frame True {
                n250 = One Button Dialog(message="호칭과 명목값 모두 입력 하세요." ("메시지")) -> ()  [unwired: 1 in, 1 out]
              }
            }
            n251 = Build Array(w409, w410, w407, w406) -> (w408:refnum<vi>[])
            n252 = call "Set State Controls.vi"("컨트롤 참조 배열 in"=w408) -> ()  [unwired: 9 in, 2 out]
          }
          frame "제거" {
            n253 = Delete From Array(array=w492, index (row)=w491) -> (array with subset deleted=w490:string[][])  [unwired: 2 in, 1 out]
            n254 = property on="시험분동" class="MCListbox (엄격한)"(error in=w494, "ItemNames"=w490) -> (error out=w493:errorcluster)  [unwired: 1 in, 1 out]
          }
        }
      }
      frame "분동추가적용" {
        w506 = Cmd_Var_Data_IO."Result_Temp" ("Select")
        w529 = Cmd_Var_Data_IO."Result" ("Select")
        n255 = property on="시험분동" class="MCListbox (엄격한)"(error in=w525) -> (error out=w542:errorcluster, "ItemNames"=w498:string[][])  [unwired: 1 in, 1 out]
        n256 = control-ref of="Spec"() -> (w538:refnum<vi>)
        n257 = control-ref of="Condition"() -> (w500:refnum<vi>)
        n258 = call "Variables Data IO.vi"("Select"=Cmd_Var_Data_IO."Condition", "error in"=w542, "Data In"=w498, "Func_ext"=w524) -> ("error out"=w541:errorcluster, "Func_ext Out"=w539:string)  [unwired: 5 in, 1 out]
        n259 = control-ref of="Measured"() -> (w535:refnum<vi>)
        n260 = control-ref of="편심오차"() -> (w536:refnum<vi>)
        n261 = control-ref of="Header2"() -> (w533:refnum<vi>)
        n262 = control-ref of="X=S-T"() -> (w532:refnum<vi>)
        n263 = call "Table Initialize_2D.vi"("Table Ref"=w500, "Value"=w498, "에러 입력"=w541) -> ("에러 출력"=w540:errorcluster)  [unwired: 6 in, 2 out]
        n264 = call "STD Cal Data_etc.vi"("error in"=w540, "Func_ext"=w539) -> ("error out"=w520:errorcluster, "Data Out"=w497:string[][], "Func_ext Out"=w521:string)  [unwired: 5 in, 2 out]
        n265 = Build Array(w535, w536, w533, w532) -> (w534:refnum<vi>[])
        n266 = call "Variables Data IO.vi"("Select"=Cmd_Var_Data_IO."Spec Temp", "error in"=w520, "Func_ext"=w521) -> ("error out"=w517:errorcluster, "Data Out"=w495:string[][], "Func_ext Out"=w496:string)  [unwired: 6 in]
        n267 = call "Set State Controls.vi"("활성화 (F)"=TRUE, "컨트롤 참조 배열 in"=w534) -> ()  [unwired: 8 in, 2 out]
        n268 = call "Get Spec.vi"("NumRows"=u32 28, "Spec in"=w495, "Spec Ref."=w538, "error in"=w517, "Condition in"=w498, "Resolution in"=w497, "Func_ext"=w496) -> ("error out"=w516:errorcluster, "Data Out"=w501:string[][], "Func_ext Out"=w519:string)  [unwired: 2 out]
        n269 = call "Variables Data IO.vi"("Select"=Cmd_Var_Data_IO."CMC Default", "error in"=w516, "Func_ext"=w519) -> ("error out"=w515:errorcluster, "Data Out"=w522:string[][], "Func_ext Out"=w518:string)  [unwired: 6 in]
        n270 = call "Match_CMC.vi"("CMC IN"=w522, "error in"=w515, "Condition IN"=w501, "Func_ext"=w518) -> ("error out"=w531:errorcluster, "Func_ext out"=w530:string)  [unwired: 4 in, 2 out]
        n271 = Index Array(array=w498, index (col)=0 ("비활성화된 인덱스 (열)")) -> (element=w503:string[])  [unwired: 1 in]
        n272 = call "Variables Data IO.vi"("Select"=w529, "error in"=w531, "Func_ext"=w530) -> ("error out"=w510:errorcluster, "Data Out"=w509:string[][], "Func_ext Out"=w508:string)  [unwired: 6 in]
        n273 = call "Variables Data IO.vi"("Select"=w506, "error in"=w510, "Func_ext"=w508) -> ("error out"=w502:errorcluster, "Data Out"=w505:string[][], "Func_ext Out"=w507:string)  [unwired: 6 in]
        n274 = for {
          tunnel: w498 -> [w559] mode=indexing
          tunnel: w509 -> [w556]
          shift-right: [w555] -> w527
          shift-left: string[][] [] -> [w553]
          tunnel: [w549] -> w512 mode=indexing
          tunnel: w505 -> [w548]
          tunnel: w503 -> [w547]
          i -> [w550]
          n275 = Index Array(array=w559) -> (element=w546:string)  [unwired: 1 in]
          n276 = Index Array(array=w556) -> (element=w558:string[])  [unwired: 2 in]
          n277 = Search 1D Array(1D array=w547, element=w546) -> (index of element=w545:i32)  [unwired: 1 in]
          n278 = Search 1D Array(1D array=w558, element=w546) -> (index of element=w557:i32)  [unwired: 1 in]
          n279 = case shown="-1" w557 {
            selector: w557 -> [w564 _]
            tunnel: w556 -> [w566 _]
            tunnel: [w565 w569] -> w554
            tunnel: w546 -> [_ w570]
            tunnel: [w560 string[] ["", "", "", "", ""]] -> w549
            tunnel: w548 -> [w562 _]
            tunnel: w545 -> [w561 _]
            frame Default {
              n280 = Index Array(array=w562, index (row)=w561) -> (element=w560:string[])  [unwired: 1 in]
              n281 = Delete From Array(array=w566, length=3 ("길이"), index (col)=w564) -> (deleted portion=w565:string[][])  [unwired: 1 in, 1 out]
            }
            frame -1 {
              w571 = 0 ("인덱스 (행)")
              n282 = Replace Array Subset(array=string[][] [["", "", ""], ["", "", ""], ["", "", ""], ["", "", ""], ["", "", ""], ["", "", ""], ["", "", ""], ["", "", ""]], new element=w570, index (row)=w571, index (col)=w571) -> (w569:string[][])
            }
          }
          n283 = Multiply(x=w550, y=3) -> (x*y=w551:i32)
          n284 = Insert Into Array(array=w553, index (col)=w551, new element=w554) -> (w555:string[][])  [unwired: 1 in]
        }
        n285 = call "Variables Data IO.vi"("Select"=w506, "error in"=w502, "Data In"=w512, "Func_ext"=w507) -> ("error out"=w513:errorcluster, "Func_ext Out"=w511:string)  [unwired: 5 in, 1 out]
        n286 = call "Variables Data IO.vi"("Select"=w529, "error in"=w513, "Data In"=w527, "Func_ext"=w511) -> ("error out"=w514:errorcluster)  [unwired: 5 in, 2 out]
      }
      frame "분동등급변경" {
        w578 = Cmd_Var_Data_IO."Result_Temp" ("Select")
        n287 = local read "시험분동"() -> (w573:i32)
        n288 = local read "분동등급"() -> (w574:string)
        n289 = call "Variables Data IO.vi"("Select"=w578, "error in"=w582, "Func_ext"=w581) -> ("error out"=w580:errorcluster, "Data Out"=w576:string[][], "Func_ext Out"=w579:string)  [unwired: 6 in]
        n290 = control-ref of="Measured"() -> (w589:refnum<vi>)
        n291 = control-ref of="편심오차"() -> (w590:refnum<vi>)
        n292 = control-ref of="Header2"() -> (w591:refnum<vi>)
        n293 = control-ref of="X=S-T"() -> (w592:refnum<vi>)
        n294 = call <vilib>:"Trim Whitespace.vi"("string"=w574) -> ("trimmed string"=w587:string)  [unwired: 1 in]
        n295 = case shown="참" "일괄\n변경" {
          tunnel: w576 -> [w596 w605]
          tunnel: [w595 w604] -> w575
          tunnel: w574 -> [w594 w602]
          tunnel: w573 -> [_ w601]
          frame True {
            n296 = for {
              tunnel: w596 -> [w600] mode=indexing
              tunnel: w594 -> [w599]
              tunnel: [w598] -> w595 mode=indexing
              n297 = Replace Array Subset(array=w600, new element=w599, index=2 ("인덱스")) -> (w598:string[])
            }
          }
          frame False {
            n298 = Replace Array Subset(array=w605, new element=w602, index (row)=w601, index (col)=2 ("인덱스")) -> (w604:string[][])
          }
        }
        n299 = Empty String/Path?(string/path=w587) -> (empty?=w586:bool)
        n300 = Build Array(w589, w590, w591, w592) -> (w588:refnum<vi>[])
        n301 = Select(t=FALSE, s=w586, f=TRUE) -> (s? t:f=w583:bool)
        n302 = call "Set State Controls.vi"("활성화 (F)"=w583, "컨트롤 참조 배열 in"=w588) -> ()  [unwired: 8 in, 2 out]
        n303 = call "Variables Data IO.vi"("Select"=w578, "error in"=w580, "Data In"=w575, "Func_ext"=w579) -> ("error out"=w577:errorcluster)  [unwired: 5 in, 2 out]
      }
    }
  }
  n304 = Release Queue(queue=w10, error in (no error)=w11) -> (error out=w8:errorcluster)  [unwired: 1 in, 2 out]
  n305 = Merge Errors(w9, w8) -> (→"에러 출력":errorcluster)
